vi "Avocent_value_switches.vi"(11 "Power indicator 2":bool[](array[boolean])=[FALSE, TRUE, TRUE, FALSE, TRUE, TRUE, FALSE, FALSE, TRUE, FALSE, TRUE, TRUE, TRUE, TRUE, TRUE, TRUE, FALSE, FALSE, FALSE, FALSE, FALSE, FALSE, FALSE, FALSE, FALSE, FALSE, FALSE, FALSE, FALSE, FALSE, FALSE, FALSE] caption="Power indicator") -> (3 "spreadsheet string":string="0110110010111111")   [LabVIEW 2020]
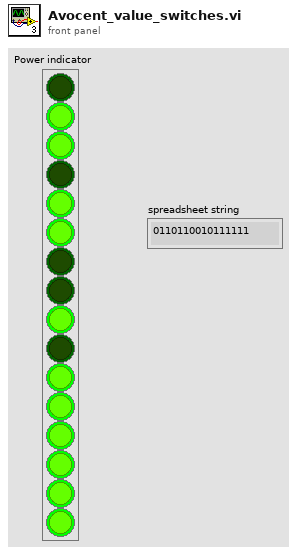
[diagram p1: front panel]
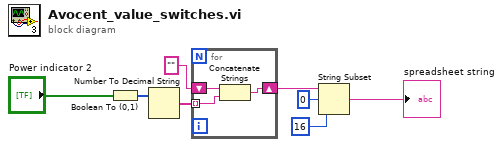
[diagram p0: block diagram]
diagram:
  n1 = Boolean To (0,1)(Boolean="Power indicator 2") -> (0, 1=w8:i16[])
  n2 = Number To Decimal String(number=w8) -> (decimal integer string=w6:string[])  [unwired: 1 in]
  n3 = for {
    tunnel: w6 -> [w9] mode=indexing
    shift-right: [w11] -> w4
    shift-left: "" -> [w10]
    n4 = Concatenate Strings(w10, w9) -> (w11:string)
  }
  n5 = String Subset(string=w4, offset (0)=0, length (rest)=16 ("length (rest)")) -> (substring=→"spreadsheet string":string)
